vi "Timer_GetElapsedTime.vi"(8 "error in (no error)":errorcluster, 11 "Timer Data Reference (in)":refnum<data-value>) -> (0 "error out":errorcluster, 1 "Is Time Elapsed?":bool, 2 "Time Elapsed (s)":dbl, 3 "Timer Data Reference (out)":refnum<data-value>)   [LabVIEW 2024]
doc: "Gets the Elapsed Time and if Total Elapsed.\n\n--------\nPaulo Rossi\nprossi@aurumautomation.ca\n©2024 Aurum Automation Inc.\nOpen-Sourced per GNU GPL v3\n\nYou should have received a copy of the GNU General Public License along with this program. If not, see <https://www.gnu.org/licenses/>."
uses:
  Timer_Data.ctl
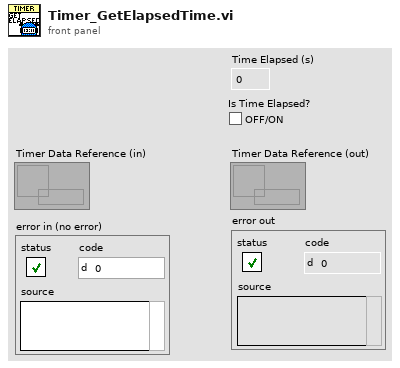
[diagram p1: front panel]
types:
  T1 = typedef "Timer_Data.ctl" = cluster{"Starting Time":dbl, "Time Elapsed (s)":dbl, "Is Time Elapsed?":bool, "Target Time (s)":dbl, "Pause Start Time":dbl, "Pause Elapsed Time":dbl, "Is Paused?":bool, "Cumulative Paused Time":dbl}
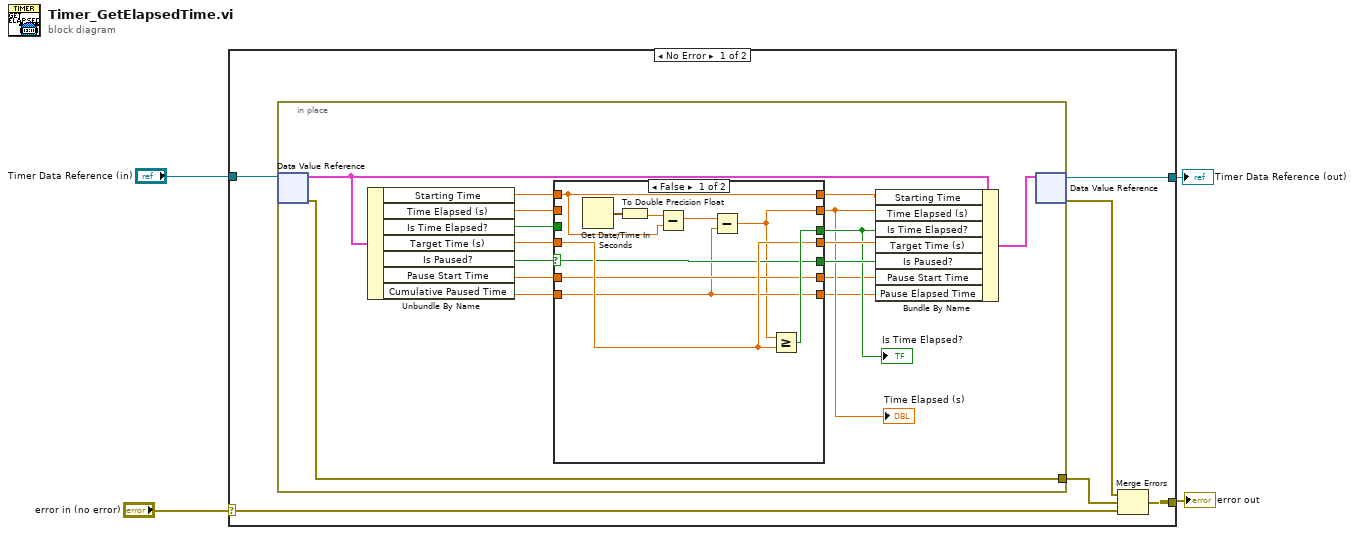
[diagram p0: block diagram]
diagram:
  n1 = case shown="No Error" "error in (no error)" {
    selector: "error in (no error)" -> [w5 w46]
    tunnel: [w8 w46] -> w3
    tunnel: "Timer Data Reference (in)" -> [w10 w45]
    tunnel: [w9 w45] -> w1
    frame No Error {
      n2 = in-place {
        in-place-border: [w26] -> w6
        n3 = in-place-dvr #1(w10) -> (w25:T1, w26:errorcluster)
        n4 = Unbundle By Name(w25) -> ("Starting Time"=w17:dbl, "Time Elapsed (s)"=w18:dbl, "Is Time Elapsed?"=w19:bool, "Target Time (s)"=w22:dbl, "Is Paused?"=w24:bool, "Pause Start Time"=w12:dbl, "Cumulative Paused Time"=w14:dbl)
        n5 = case shown="False" w24 {
          selector: w24 -> [w34 w42]
          tunnel: w17 -> [w31 w40]
          tunnel: [w28 w41] -> w15
          tunnel: [w36 w43] -> w20
          tunnel: w22 -> [w35 w44]
          tunnel: [w31 w40] -> w16
          tunnel: w18 -> [_ w41]
          tunnel: [w35 w44] -> w21
          tunnel: w19 -> [_ w43]
          tunnel: [w34 w42] -> w23
          tunnel: w14 -> [w29 w39]
          tunnel: [w29 w39] -> w13
          tunnel: w12 -> [w33 w38]
          tunnel: [w33 w38] -> w11
          frame False {
            n6 = Get Date/Time In Seconds() -> (seconds since 1Jan1904=w37:timestamp)
            n7 = To Double Precision Float(number=w37) -> (double precision float=w32:dbl)
            n8 = Subtract(x=w32, y=w31) -> (x-y=w30:dbl)
            n9 = Subtract(x=w30, y=w29) -> (x-y=w28:dbl)
            n10 = Greater Or Equal?(x=w28, y=w35) -> (x >= y?=w36:bool)
          }
          frame True {
          }
        }
        "Is Time Elapsed?" <- w20
        "Time Elapsed (s)" <- w15
        n11 = Bundle By Name(cluster=w25, "Starting Time"=w16, "Time Elapsed (s)"=w15, "Is Time Elapsed?"=w20, "Target Time (s)"=w21, "Is Paused?"=w23, "Pause Start Time"=w11, "Pause Elapsed Time"=w13) -> (w27:T1)
        n12 = in-place-dvr #1(w27) -> (w9:refnum<data-value>, w7:errorcluster)
      }
      n13 = Merge Errors(w7, w6, w5) -> (w8:errorcluster)
    }
    frame Error {
    }
  }
  "error out" <- w3
  "Timer Data Reference (out)" <- w1
